vi "Write Poll Rate.vi"(8 "error in (no error)":cluster{"状态":bool, "代码":i32, "源":string} caption="错误输入（无错误）", 10 "轮询速率":i64, 11 "水位控制器输入":refnum<class "Timed Loop Actor.lvclass">) -> (0 "error out":cluster{"状态":bool, "代码":i32, "源":string} caption="错误输出", 3 "水位控制器输出":refnum<class "Timed Loop Actor.lvclass">)   [LabVIEW 2015, in "Timed Loop Actor.lvlib" / "Timed Loop Actor.lvclass"]
doc: "设置循环每次迭代的时间间隔。"
uses:
  Timed Loop Actor.lvclass
  Timed Loop Actor.lvclass/Timed Loop Actor.ctl
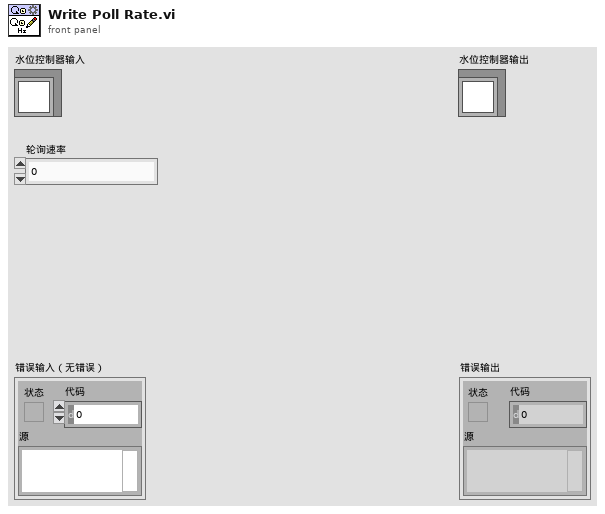
[diagram p1: front panel]
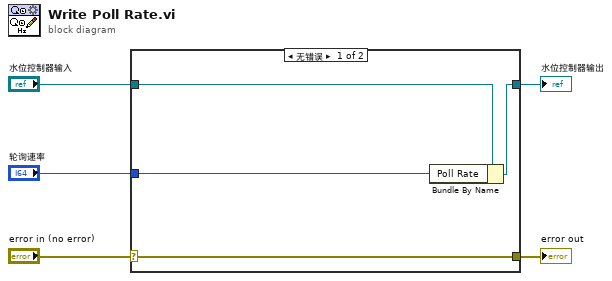
[diagram p0: block diagram]
diagram:
  n1 = case shown="无错误" "error in (no error)" {
    selector: "error in (no error)" -> [w9 w10]
    tunnel: [w9 w10] -> w4
    tunnel: [w7 w11] -> w2
    tunnel: "水位控制器输入" -> [w8 w11]
    tunnel: "轮询速率" -> [w6 _]
    frame No Error {
      n2 = Bundle By Name(cluster=w8, "Poll Rate"=w6) -> (w7:refnum<class "Timed Loop Actor.lvclass">)
    }
    frame Error {
    }
  }
  "error out" <- w4
  "水位控制器输出" <- w2
